vi "Get_Each_channel_reference_samplingdata.vi"(0 "SPU":refnum<k24>, 1 "STSProcess.ILSTS":refnum<k24>, 2 "Refdata_struct":refnum<k24>[](array[refnum]), 5 "Ref_monitordata_struct":refnum<k24>[](array[refnum]), 7 "MPM":refnum<k24>[](array[refnum]), 9 "ChannelNumber":i32, 11 "错误输入（无错误）":errorcluster, 13 "SlotNumber":i32, 14 "MPMNumber":i32) -> (6 "ILSTS out":refnum<k24>, 15 "error out":errorcluster)   [LabVIEW 2017]
doc: "Get logging reference data & add in"
uses:
  D:/test/ILSTS/LV_IL_Sample/DLL/STSProcess.dll
  DLL/STSProcess.dll
  D:/test/ILSTS/LV_IL_Sample/DLL/InstrumentDLL.dll
  DLL/InstrumentDLL.dll
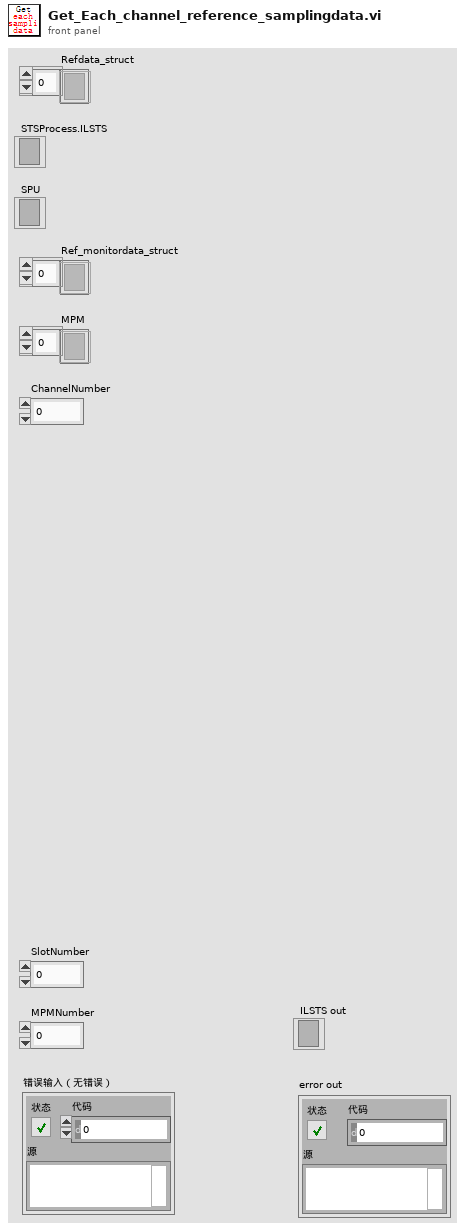
[diagram p1: front panel]
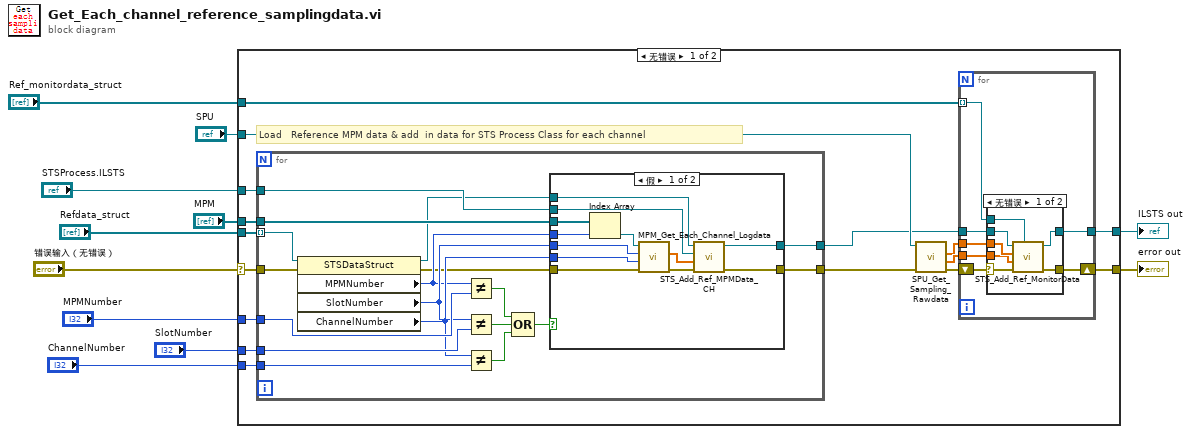
[diagram p0: block diagram]
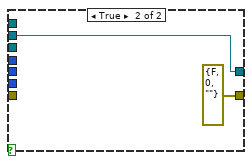
[diagram p3: hidden frame]
diagram:
  n1 = case shown="无错误" "错误输入（无错误）" {
    selector: "错误输入（无错误）" -> [w15 w77]
    tunnel: "STSProcess.ILSTS" -> [w13 w76]
    tunnel: "Ref_monitordata_struct" -> [w24 _]
    tunnel: "SPU" -> [w23 _]
    tunnel: "MPM" -> [w21 _]
    tunnel: "ChannelNumber" -> [w20 _]
    tunnel: "SlotNumber" -> [w19 _]
    tunnel: "MPMNumber" -> [w18 _]
    tunnel: "Refdata_struct" -> [w17 _]
    tunnel: [w16 w77] -> w3
    tunnel: [w14 w76] -> w1
    frame No Error {
      # "Load　Reference MPM data & add  in data for STS Process Class for each channel"
      n2 = for {
        tunnel: w17 -> [w49] mode=indexing
        tunnel: w18 -> [w61]
        tunnel: w19 -> [w60]
        tunnel: w20 -> [w59]
        tunnel: w21 -> [w52]
        tunnel: w13 -> [w50]
        tunnel: [w48] -> w22
        tunnel: w15 -> [w46]
        tunnel: [w44] -> w12
        n3 = property on="属性节点" class="STSDataStruct"(reference=w49, error in=w46) -> (reference out=w45:refnum<k24>, error out=w47:errorcluster, "MPMNumber"=w51:i32, "SlotNumber"=w54:i32, "ChannelNumber"=w53:i32)
        n4 = Not Equal?(x=w51, y=w61) -> (x != y?=w58:bool)
        n5 = Not Equal?(x=w54, y=w60) -> (x != y?=w57:bool)
        n6 = Not Equal?(x=w53, y=w59) -> (x != y?=w56:bool)
        n7 = Compound Arithmetic op=OR ("复合运算")(w58, w57, w56) -> (w55:bool)
        n8 = case shown="假" w55 {
          tunnel: w54 -> [w73 _]
          tunnel: w53 -> [w72 _]
          tunnel: w52 -> [w71 _]
          tunnel: w51 -> [w69 _]
          tunnel: w50 -> [w68 w74]
          tunnel: w45 -> [w67 _]
          tunnel: [w64 errorcluster {"status"=FALSE, "code"=0, "source"=""} ("错误输出")] -> w48
          tunnel: w47 -> [w63 _]
          tunnel: [w62 w74] -> w44
          frame False {
            n9 = Index Array(array=w71, index=w69) -> (element=w70:refnum<k24>)
            n10 = call "MPM_Get_Each_Channel_Logdata.vi"("error in (no error)"=w63, "channelNumber"=w72, "moduleNumber"=w73, ".NET Reference in"=w70) -> ("error out"=w65:errorcluster, "data out"=w66:sgl[])  [unwired: 5 in, 1 out]
            n11 = call "STS_Add_Ref_MPMData_CH.vi"("错误输入（无错误）"=w65, "data"=w66, "STSProcess.ILSTS"=w68, "Setting"=w67) -> ("错误输出"=w64:errorcluster, "ILSTS"=w62:refnum<k24>)  [unwired: 6 in]
          }
          frame True {
          }
        }
      }
      n12 = call "SPU_Get_Sampling_Rawdata.vi"("错误输入（无错误）"=w22, "SPU"=w23) -> ("error out"=w25:errorcluster, "monitor"=w27:sgl[], "trigger"=w26:sgl[])  [unwired: 5 in, 1 out]
      n13 = for {
        tunnel: w24 -> [w33] mode=indexing
        tunnel: w12 -> [w34]
        tunnel: w26 -> [w32]
        tunnel: w27 -> [w31]
        shift-right: [w29] -> w16
        shift-left: w25 -> [w30]
        tunnel: [w28] -> w14
        n14 = case shown="无错误" w30 {
          selector: w30 -> [w37 w43]
          tunnel: w34 -> [w41 w42]
          tunnel: w33 -> [w40 _]
          tunnel: w32 -> [w39 _]
          tunnel: w31 -> [w38 _]
          tunnel: [w36 w43] -> w29
          tunnel: [w35 w42] -> w28
          frame No Error {
            n15 = call "STS_Add_Ref_MonitorData.vi"("setting"=w40, "错误输入（无错误）"=w37, "monitorData"=w38, "triggerIndex"=w39, "STSProcess.ILSTS"=w41) -> ("错误输出"=w36:errorcluster, "ILSTS out"=w35:refnum<k24>)  [unwired: 5 in]
          }
          frame Error {
          }
        }
      }
    }
    frame Error {
    }
  }
  "error out" <- w3
  "ILSTS out" <- w1
